vi "Close_Instr.vi"(8 "error in (no error)":errorcluster caption="entrée d'erreur (pas d'erreur)", 11 "Class Relay_Board en entrée":refnum<class "Class Instrument UART.lvclass">) -> (0 "error out":errorcluster caption="sortie d'erreur", 3 "Class Relay_Board en Sortie":refnum<class "Class Instrument UART.lvclass">)   [LabVIEW 2020, in "Library Instrument & Equipement.lvlib" / "Library Instruments.lvlib" / "Class Instrument UART.lvclass"]
uses:
  Class Instrument UART.lvclass
  Class Instrument UART.lvclass/Class Instrument UART.ctl
  UART/UART (Default)/Class UART (Default).lvclass
  Instrument (Default)/Class Instrument (Default).lvclass
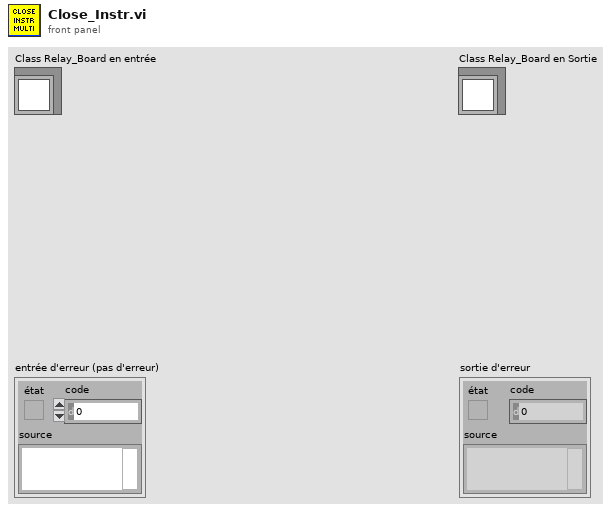
[diagram p1: front panel]
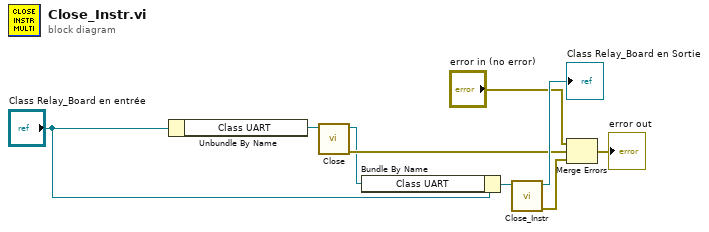
[diagram p0: block diagram]
diagram:
  n1 = Unbundle By Name("Class Relay_Board en entrée") -> ("Class UART"=w2:refnum<class "Class UART (Default).lvclass">)
  n2 = call-dynamic "Close.vi"("Class UART (Default) en entrée"=w2) -> ("error out"=w3:errorcluster, "Class UART (Default) en sortie"=w1:refnum<class "Class UART (Default).lvclass">)  [unwired: 9 in]
  n3 = Bundle By Name(cluster="Class Relay_Board en entrée", "Class UART"=w1) -> (w7:refnum<class "Class Instrument UART.lvclass">)
  n4 = call-parent "Close_Instr.vi"("Class Instrument (Default) en entrée"=w7) -> ("error out"=w5:errorcluster, "Class Instrument (Default) en sortie"=→"Class Relay_Board en Sortie":refnum<class "Class Instrument UART.lvclass">)  [unwired: 9 in]
  n5 = Merge Errors("error in (no error)", w3, w5) -> (→"error out":errorcluster)
